vi "PMS7003_Driver.vi"() -> ()   [LabVIEW 2019]
uses:
  C:/Program Files (x86)/National Instruments/LabVIEW 2019/examples/Instrument IO/Serial/support/Serial - Settings.ctl
  C:/Program Files (x86)/National Instruments/LabVIEW 2019/examples/Instrument IO/Serial/support/Serial - XON-XOFF Characters.ctl
  C:/Program Files (x86)/National Instruments/LabVIEW 2019/examples/Instrument IO/Serial/support/Serial - ASCII Characters.ctl
  <vilib>/Instr/_visa.llb/VISA Configure Serial Port (Instr).vi
panel:
  out "x = y?":bool
  out "Check Sum":u32
  out "Data":u16[](array[numeric])
  in  "Read Count 2":u32=1000
  in  "Command 2":string="*IDN?"
  in  "Stop 2":bool
  in  "Write 2":bool
  in  "Termination Character":u8=10 format="%.0x"
  in  "End Write on Termination Character?":bool=TRUE
  in  "VISA resource name":refnum<visa-resource-name>="COM4"
  in  "XON/XOFF Characters":T1={"XON"=enum."DC1", "XOFF"=enum."DC3"}
  in  "Serial Settings":T3={"baud rate"=9600, "data bits"=8, "parity"=enum."None", "stop bits"=10, "flow control"=0} {"flow control" items=["None"=0, "XON/XOFF"=1, "RTS/CTS"=2, "DTR/DSR"=4]; "stop bits" items=["1.0"=10, "1.5"=15, "2.0"=20]; "data bits" min=5 max=8 step=1; "baud rate" items=["75"=75, "110"=110, "134"=134, "150"=150, "300"=300, "600"=600, "1200"=1200, "1800"=1800, "2400"=2400, "4800"=4800, "7200"=7200, "9600"=9600, "14400"=14400, "19200"=19200, "28800"=28800, "38400"=38400, "56000"=56000, "57600"=57600, "115200"=115200, "128000"=128000, "230400"=230400]}
  in  "End Read on Termination Character?":bool=TRUE
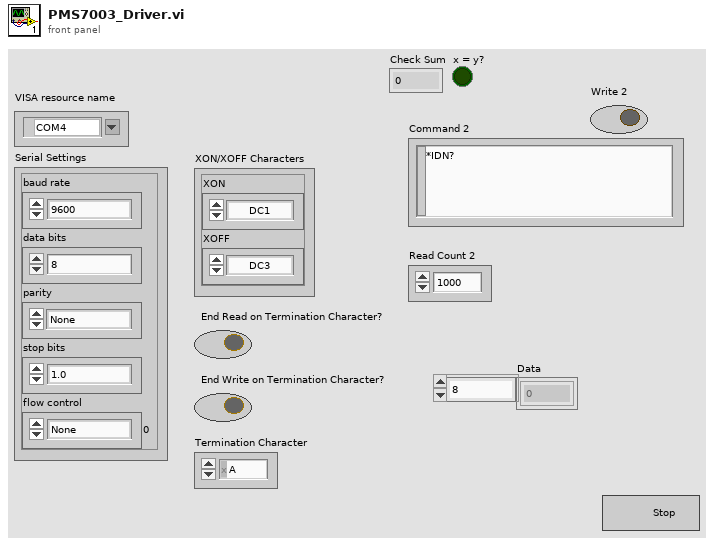
[diagram p1: front panel]
types:
  T1 = typedef "Serial - XON-XOFF Characters.ctl" = cluster{"XON":T2, "XOFF":T2}
  T2 = typedef "Serial - ASCII Characters.ctl" = enum16{"NUL", "SOH", "STX", "ETX", "EOT", "ENQ", "ACK", "BEL", "BS", "HT", "LF", "VT", "FF", "CR", "SO", "SI", "DLE", "DC1", "DC2", "DC3", "DC4", "NAK", "SYN", "ETB", "CAN", "EM", "SUB", "ESC", "FS", "GS", "RS", "US", "SP", "!", "\"", "#", "$", "%", "&", "'", "(", ")", "*", "+", ",", "- (-)", ".", "/", "0", "1", "2", "3", "4", "5", "6", "7", "8", "9", ":", ";", "<", "=", ">", "?", "@", "A", "B", "C", "D", "E", "F", "G", "H", "I", "J", "K", "L", "M", "N", "O", "P", "Q", "R", "S", "T", "U", "V", "W", "X", "Y", "Z", "[", "\\", "]", "^", "_", "`", "a", "b", "c", "d", "e", "f", "g", "h", "i", "j", "k", "l", "m", "n", "o", "p", "q", "r", "s", "t", "u", "v", "w", "x", "y", "z", "{", "|", "}", "~"}
  T3 = typedef "Serial - Settings.ctl" = cluster{"baud rate":u32, "data bits":u16, "parity":enum16{"None", "Odd", "Even", "Mark", "Space"}, "stop bits":u16, "flow control":u16}
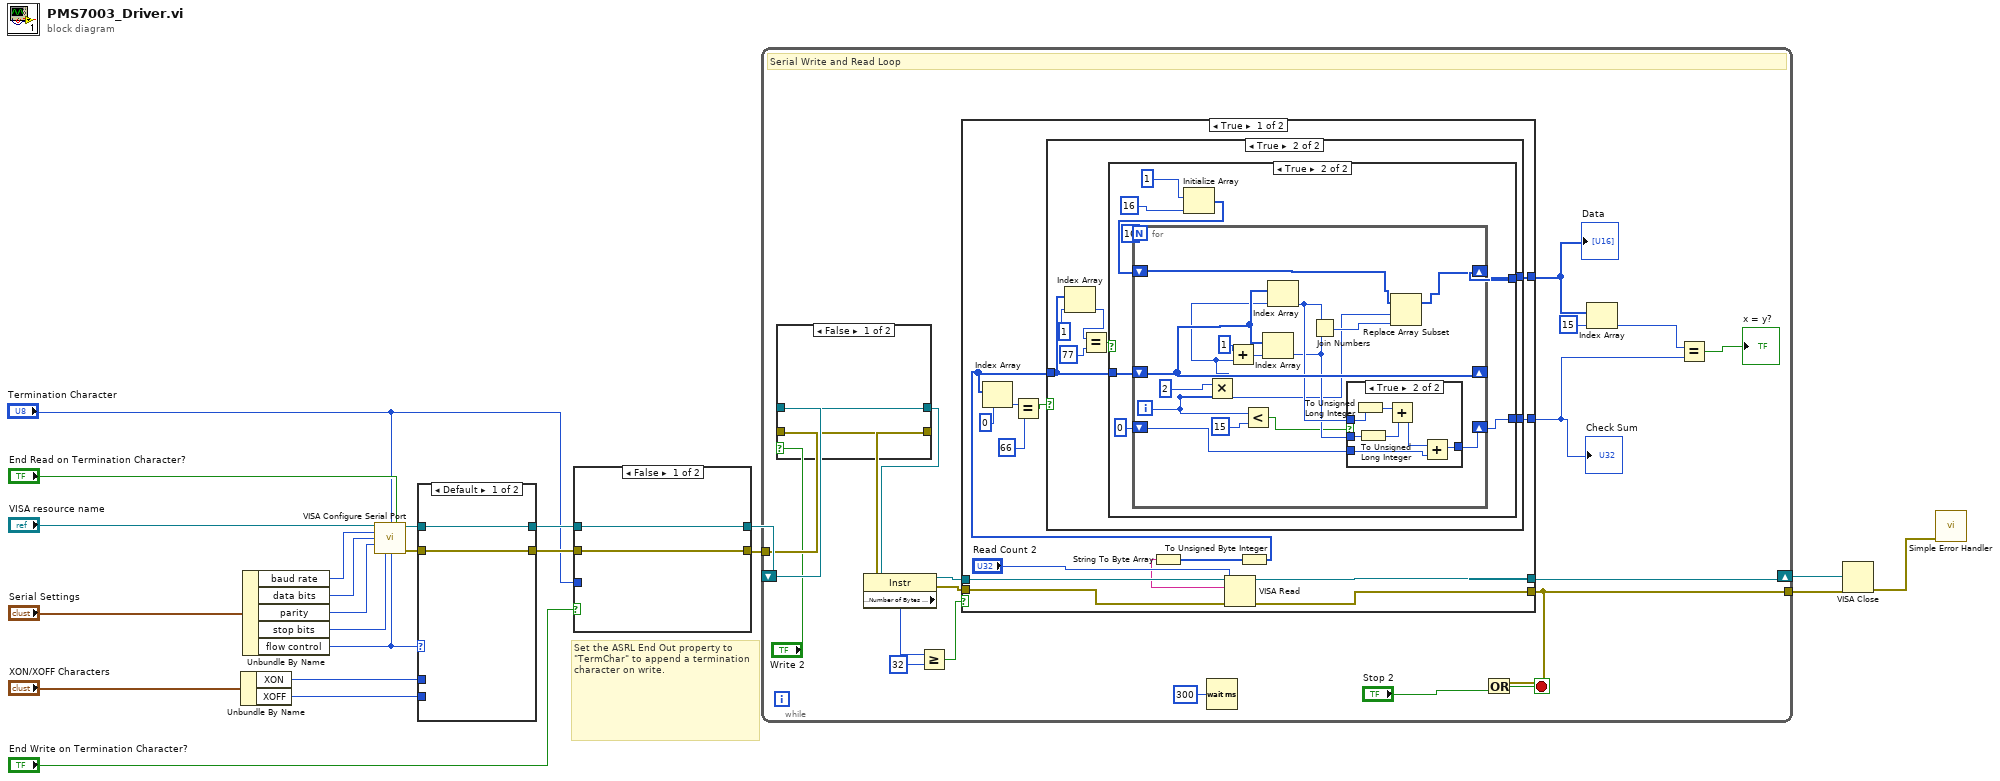
[diagram p0: block diagram]
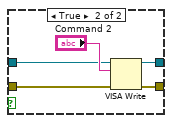
[diagram p2: hidden frame]
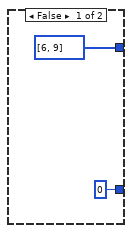
[diagram p3: hidden frame]
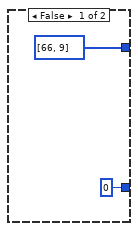
[diagram p4: hidden frame]
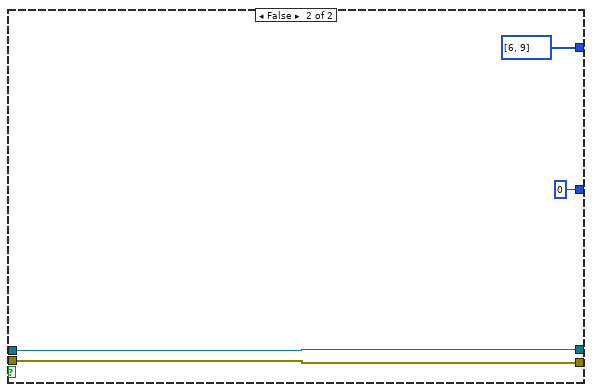
[diagram p6: hidden frame]
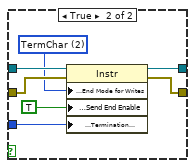
[diagram p7: hidden frame]
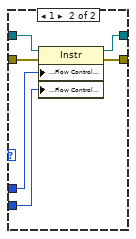
[diagram p8: hidden frame]
diagram:
  # "Set the ASRL End Out property to \"TermChar\" to append a termination character on write."
  n1 = Unbundle By Name("XON/XOFF Characters") -> ("XON"=w10:T2, "XOFF"=w9:T2)
  n2 = Unbundle By Name("Serial Settings") -> ("baud rate"=w15:u32, "data bits"=w16:u16, "parity"=w17:enum16{"None", "Odd", "Even", "Mark", "Space"}, "stop bits"=w18:u16, "flow control"=w11:u16)
  n3 = call-poly "VISA Configure Serial Port"("VISA resource name"="VISA resource name", "termination char\n(0xA = '\\n' = LF)"="Termination Character", "Enable Termination\nChar (T)"="End Read on Termination Character?", "baud rate (9600)"=w15, "data bits (8)"=w16, "parity (0:none)"=w17, "stop bits (10: 1 bit)"=w18, "flow control (0:none)"=w11) -> ("VISA resource name out"=w19:refnum<visa-resource-name>, "error out"=w20:errorcluster)  [unwired: 2 in, 4 out]
  n4 = case shown="Default" w11 {
    tunnel: [w23 w30] -> w8
    tunnel: [w24 w29] -> w7
    tunnel: w20 -> [w23 w28]
    tunnel: w19 -> [w24 w27]
    tunnel: w10 -> [_ w26]
    tunnel: w9 -> [_ w25]
    frame Default {
    }
    frame 1 {
      n5 = property class="Instr"(reference=w27, error in=w28, "Serial Settings:Flow Control XON Character"=w26, "Serial Settings:Flow Control XOFF Character"=w25) -> (reference out=w29:refnum<visa-resource-name>, error out=w30:errorcluster)
    }
  }
  n6 = case shown="False" "End Write on Termination Character?" {
    tunnel: w7 -> [w31 w39]
    tunnel: w8 -> [w32 w38]
    tunnel: [w31 w37] -> w4
    tunnel: [w32 w36] -> w3
    tunnel: "Termination Character" -> [_ w34]
    frame False {
    }
    frame True {
      w35 = u16 2 items=["None", "LastBit", "TermChar", "Break"] ("Serial Settings:Serial End Mode for Writes")
      n7 = property class="Instr"(reference=w39, error in=w38, "Serial Settings:End Mode for Writes"=w35, "Message Based Settings:Send End Enable"=TRUE, "Message Based Settings:Termination Character"=w34) -> (reference out=w37:refnum<visa-resource-name>, error out=w36:errorcluster)
    }
  }
  n8 = while {
    shift-right: [w59] -> w2
    shift-left: w4 -> [w58]
    tunnel: w3 -> [w57]
    tunnel: [w54] -> w1
    stop <- w55 stop-if-true
    # "Serial Write and Read Loop"
    n9 = case shown="False" "Write 2" {
      tunnel: w58 -> [w61 w65]
      tunnel: w57 -> [w60 w64]
      tunnel: [w61 w63] -> w46
      tunnel: [w60 w62] -> w45
      frame False {
      }
      frame True {
        n10 = VISA Write(VISA resource name=w65, write buffer="Command 2", error in (no error)=w64) -> (VISA resource name out=w63:refnum<visa-resource-name>, error out=w62:errorcluster)  [unwired: 1 out]
      }
    }
    n11 = property class="Instr"(reference=w46, error in=w45) -> (reference out=w44:refnum<visa-resource-name>, error out=w43:errorcluster, "Serial Settings:Number of Bytes at Serial Port"=w42:u32)
    n12 = Greater Or Equal?(x=w42, y=u32 32) -> (x >= y?=w40:bool)
    n13 = case shown="True" w40 {
      tunnel: [w78 w126] -> w59
      tunnel: w44 -> [w80 w126]
      tunnel: [w76 w125] -> w54
      tunnel: w43 -> [w79 w125]
      tunnel: [w73 u16[] [6, 9]] -> w51
      tunnel: [w67 u32 0] -> w49
      frame True {
        n14 = VISA Read(VISA resource name=w80, byte count="Read Count 2", error in (no error)=w79) -> (VISA resource name out=w78:refnum<visa-resource-name>, read buffer=w75:string, error out=w76:errorcluster)  [unwired: 1 out]
        n15 = String To Byte Array(string=w75) -> (unsigned byte array=w74:u8[])
        n16 = To Unsigned Byte Integer(number=w74) -> (unsigned 8bit integer=w68:u8[])
        n17 = Index Array(array=w68, index=0) -> (element=w71:u8)
        n18 = Equal?(x=w71, y=u8 66) -> (x = y?=w69:bool)
        n19 = case shown="True" w69 {
          tunnel: w68 -> [_ w88]
          tunnel: [u16[] [6, 9] w89] -> w73
          tunnel: [u32 0 w83] -> w67
          frame False {
          }
          frame True {
            n20 = Index Array(array=w88, index=1) -> (element=w85:u8)
            n21 = Equal?(x=w85, y=u8 77) -> (x = y?=w84:bool)
            n22 = case shown="True" w84 {
              tunnel: w88 -> [_ w99]
              tunnel: [u16[] [66, 9] w97] -> w89
              tunnel: [u32 0 w93] -> w83
              frame False {
              }
              frame True {
                n23 = Initialize Array(1 ("index"), 16 ("index")) -> (w96:i32[])
                n24 = for {
                  N: 16 -> [_]
                  shift-right: [w114] -> _
                  shift-left: w99 -> [w114]
                  shift-right: [w109] -> w97
                  shift-left: w96 -> [w110]
                  shift-right: [w106] -> w93
                  shift-left: u32 0 -> [w102]
                  i -> [w104]
                  n25 = Multiply(x=2, y=w104) -> (x*y=w100:i32)
                  n26 = Add(x=1, y=w100) -> (x+y=w101:i32)
                  n27 = Less?(x=w104, y=15) -> (x < y?=w105:bool)
                  n28 = Index Array(array=w114, index=w101) -> (element=w107:u8)
                  n29 = Index Array(array=w114, index=w100) -> (element=w108:u8)
                  n30 = Join Numbers(hi=w108, lo=w107) -> ((hi.lo)=w111:u16)
                  n31 = case shown="True" w105 {
                    tunnel: w108 -> [_ w118]
                    tunnel: w107 -> [_ w117]
                    tunnel: [w115 w121] -> w106
                    tunnel: w102 -> [w115 w116]
                    frame False {
                    }
                    frame True {
                      n32 = To Unsigned Long Integer(number=w118) -> (unsigned 32bit integer=w119:u32)
                      n33 = To Unsigned Long Integer(number=w117) -> (unsigned 32bit integer=w120:u32)
                      n34 = Add(x=w119, y=w120) -> (x+y=w122:u32)
                      n35 = Add(x=w122, y=w116) -> (x+y=w121:u32)
                    }
                  }
                  n36 = Replace Array Subset(array=w110, new element=w111, index=w104) -> (w109:i32[])
                }
              }
            }
          }
        }
      }
      frame False {
      }
    }
    "Data" <- w51
    "Check Sum" <- w49
    n37 = Wait (ms)(milliseconds to wait=u32 300) -> ()  [unwired: 1 out]
    n38 = Or(x=w54, y="Stop 2") -> (x .or. y?=w55:bool)
    n39 = Index Array(array=w51, index=15) -> (element=w48:i32)
    n40 = Equal?(x=w48, y=w49) -> (x = y?=→"x = y?":bool)
  }
  n41 = VISA Close(VISA resource name=w2, error in (no error)=w1) -> (error out=w12:errorcluster)
  n42 = call <vilib>:"Simple Error Handler.vi"("error in (no error)"=w12) -> ()  [unwired: 1 in, 8 out]
